vi "Channels_for_Clipping_Check.vi"() -> (0 "Channel Indicies":i32[](array[numeric]))   [LabVIEW 2010]
uses:
  Controls/Inst_type.ctl
  Globals/Meas_global.vi
  Globals/Dynamic_call_global.ph.vi
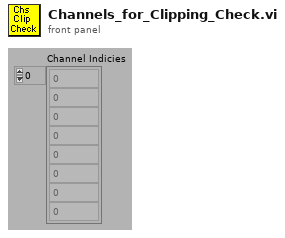
[diagram p1: front panel]
types:
  T1 = typedef "Analysis_info_cluster.ctl" = cluster{"Colour":u32, "Inst type":T2, "Inst name":string, "Symbol":string, "Code name":string, "Extra Info":string, "Inst Array":T3, "Index":i32, "Voltage Index":i32, "Extra Titles":string[], "Extra Values":string[]}
  T2 = typedef "Inst_type.ctl" = enum16{"Propeller anemometer", "Raw voltage", "Pressure Transducer", "Pitot-static tube", "Preston tube", "Hot wire", "Cross wire 1", "Cross wire 2", "Generic Linear", "Generic Polynomial", "Generic BackPoly", "Fast FID", "Thermocouple", "Cold wire", "Pulsed Wire", "LDA Vel", "LDA Tran time", "LDA Arr time"}
  T3 = typedef "Instrument_Array.ctl" = enum16{"PWA", "LDA", "Analogue"}
  T4 = typedef "Analysis_type_cluster.ctl" = cluster{"Analysis type":T5, "Indicies":i32[], "Name":string, "Inst Array":T3, "Info index":i32}
  T5 = typedef "Analysis_type_Enum.ctl" = enum16{"Slow Response", "Fast Response", "Weighted Fast Response", "Fast FID", "Weighted Fast FID", "Cross Wire", "Weighted Cross Wire", "Weighted LDA"}
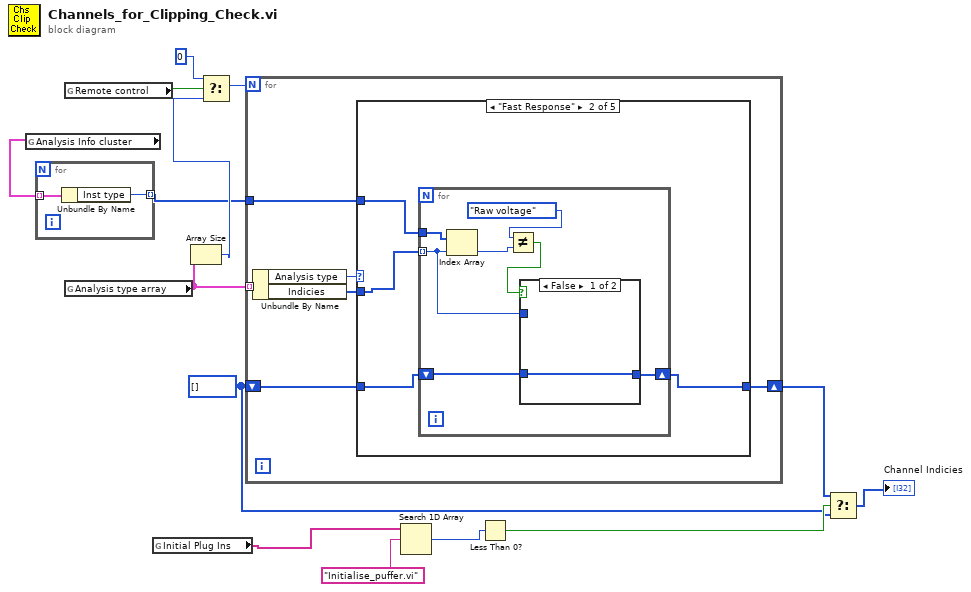
[diagram p0: block diagram]
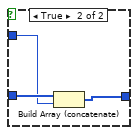
[diagram p3: hidden frame]
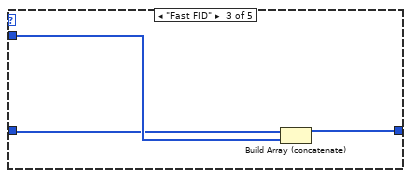
[diagram p4: hidden frame]
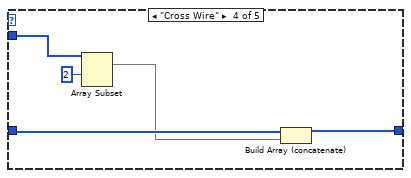
[diagram p5: hidden frame]
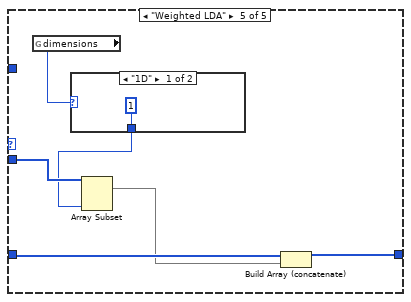
[diagram p6: hidden frame]
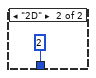
[diagram p7: hidden frame]
diagram:
  w5 = i32[] []
  n1 = global read "Meas_global.vi" "Analysis Info cluster"() -> (w2:T1[])
  n2 = for {
    tunnel: w2 -> [w16] mode=indexing
    tunnel: [w15] -> w1 mode=indexing
    n3 = Unbundle By Name(w16) -> ("Inst type"=w15:T2)
  }
  n4 = global read "Meas_global.vi" "Remote control"() -> (w12:bool)
  n5 = global read "Meas_global.vi" "Analysis type array"() -> (w14:T4[])
  n6 = global read "Dynamic_call_global.ph.vi" "Initial Plug Ins"() -> (w3:string[])
  n7 = Array Size(array=w14) -> (size(s)=w10:i32)
  n8 = Select(t=0, s=w12, f=w10) -> (s? t:f=w13:i32)
  n9 = for {
    N: w13 -> [_]
    tunnel: w14 -> [w22] mode=indexing
    shift-right: [w19] -> w6
    shift-left: w5 -> [w20]
    tunnel: w1 -> [w17]
    n10 = Unbundle By Name(w22) -> ("Analysis type"=w21:T5, "Indicies"=w18:i32[])
    n11 = case shown="\"Fast Response\"" w21 {
      tunnel: w20 -> [w23 w25 w40 w46 w52]
      tunnel: [w23 w24 w39 w45 w51] -> w19
      tunnel: w18 -> [_ w27 w41 w44 w50]
      tunnel: w17 -> [_ w26 _ _ _]
      frame "Slow Response", Default {
      }
      frame "Fast Response" {
        n12 = for {
          tunnel: w27 -> [w29] mode=indexing
          tunnel: w26 -> [w34]
          shift-right: [w28] -> w24
          shift-left: w25 -> [w30]
          n13 = Index Array(array=w34, index=w29) -> (element=w33:T2)
          n14 = Not Equal?(x=Inst_type."Raw voltage" ("element"), y=w33) -> (x != y?=w31:bool)
          n15 = case shown="False" w31 {
            tunnel: w30 -> [w35 w38]
            tunnel: w29 -> [_ w37]
            tunnel: [w35 w36] -> w28
            frame False {
            }
            frame True {
              n16 = Build Array (concatenate)(w38, w37) -> (w36:i32[])
            }
          }
        }
      }
      frame "Fast FID" {
        n17 = Build Array (concatenate)(w40, w41) -> (w39:i32[])
      }
      frame "Cross Wire" {
        n18 = Array Subset(array=w44, index=2 ("Array Index")) -> (w42:i32[])  [unwired: 1 in]
        n19 = Build Array (concatenate)(w46, w42) -> (w45:i32[])
      }
      frame "Weighted LDA" {
        n20 = global read "Meas_global.vi" "dimensions"() -> (w48:enum16{"1D", "2D"})
        n21 = case shown="\"1D\"" w48 {
          tunnel: [1 ("Array Index") 2 ("Array Index")] -> w47
          frame "1D" {
          }
          frame "2D" {
          }
        }
        n22 = Array Subset(array=w50, length=w47) -> (w49:i32[])  [unwired: 1 in]
        n23 = Build Array (concatenate)(w52, w49) -> (w51:i32[])
      }
    }
  }
  n24 = Search 1D Array(1D array=w3, element="Initialise_puffer.vi") -> (index of element=w8:i32)  [unwired: 1 out]
  n25 = Less Than 0?(x=w8) -> (x < 0?=w7:bool)
  n26 = Select(t=w6, s=w7, f=w5) -> (s? t:f=→"Channel Indicies":i32[])
